vi "pt2line.vi"() -> ()   [LabVIEW 2012]
uses:
  <vilib>/Utility/file.llb/Read From Spreadsheet File (DBL).vi
  G_VEH.vi
  G_DATA.vi
panel:
  out "XY Graph":cluster{"Y":dbl[], "Y":dbl[]}[](graph)
  out "x":dbl[](array[numeric])
  out "y":dbl[](array[numeric])
  out "all rows":dbl[][](array[numeric]) format="%0.3f"
  out "path":dbl[][](array[numeric])=[[-255.216465, -224.019097, -197.334027, -175.46223, -152.92194, -136.088512, -102.998886, -54.784189, -7.516358, 50.306778, 91.062603, 97.084713, 93.1202, 88.769951, 86.75765, 81.589658, 76.301743, 66.513984, 61.367971, 45.319341, 14.450991, -36.946592, -51.800053, -55.664715, -72.629843, -125.329123, -146.219545, -155.532572, -155.231925, -148.150396, -135.052899, -119.630627, -107.638961, -104.13624, -102.377677, -84.094956, -59.779119, -30.298412, -1.547282, 2.854327, 6.657761, 10.459174, 3.511141, -26.30694, -73.476042, -111.842628, -118.995936, -116.921215, -102.705074, -88.210666, -83.464367, -86.343257, -102.617415, -107.759916], [-500.016381, -499.568356, -491.833583, -478.953387, -483.69293, -504.762747, -532.145235, -529.336413, -503.242034, -468.920949, -416.684928, -375.565995, -317.161413, -241.087674, -176.765644, 3.050236, 189.901281, 261.392787, 293.826989, 342.636657, 363.781536, 367.66991, 386.702929, 417.645918, 425.204416, 423.95351900000003, 421.057136, 404.578929, 377.734918, 362.899426, 359.271761, 354.312176, 342.051425, 318.167906, 262.459507, 222.699763, 207.938059, 194.431872, 156.064352, 93.448286, -37.349453, -127.219275, -172.925371, -232.424698, -322.447879, -394.422916, -407.829977, -419.760997, -428.914985, -435.912385, -441.894453, -447.061864, -442.947155, -438.571904], [-0.027619159683021918, 0.03119709854315155, 0.5801517623319503, 0.22974199850915422, -0.6985990286570105, -0.9293009663449048, -0.3629416523824042, 0.4364661436108174, 0.517269626400344, 0.6407274895950754, 1.202041727338265, 1.6238751525788475, 1.6374547962778776, 1.5888610615665095, 1.592488214998328, 1.6019260023104704, 1.6167108615873471, 1.7565325957017393, 1.6632287927306733, 2.2220223320446446, 2.8894133609140376, 2.6493725961179972, 1.7654388795036573, 2.1924575664831303, -3.124456663546736, -3.1171931962117276, -2.6388223143414686, -1.6335362194597147, -1.4505762061951697, -0.6355428134884025, 0.011046092972199223, -0.8136354408991358, -1.0376420447469035, -1.5493221762811478, -1.4668097598430623, -0.7797235340435182, -0.34848317538441986, -0.6205836790536368, -1.2605695601954436, -1.5525481966917887, -1.5407853718079607, -1.5350592142675334, -1.962733401760107, -2.0504512632483882, -2.048817660019718, -2.0492416975710537, -1.9356743047027372, -0.8584952334475433, -0.48041653333810286, -0.5197456398894826, -1.5337392732156923, -2.7467198900599588, 2.6204704682047826, 1.8591507266149765], [31.173097298848553, 26.913348647230613, 25.353412697049688, 20.868729331498855, 26.441054626560174, 41.739539871153646, 44.076619004466615, 53.86765552210779, 67.2303653094776, 63.8979451122852, 40.52548790718823, 58.532660795170074, 76.19455662891659, 64.34788473882465, 179.8856712687191, 186.9251021756951, 71.86540454258034, 32.82666676125214, 50.08261037391, 35.528613596596784, 50.7421338721755, 22.084837087831545, 31.10617534511584, 16.024654359701316, 52.71297713376437, 20.954867085973486, 16.10065419017421, 26.772345178567814, 15.577706313644756, 12.693639675564514, 15.366548203355588, 17.147584175475338, 22.348948287332743, 55.733315576213904, 41.44270545761075, 27.66988575085065, 32.320665344175666, 45.701271321041276, 60.97074789973921, 130.84536386325192, 89.94342098656917, 45.428662749114835, 66.37743516511998, 101.63171501074622, 81.55665134233071, 15.194986170689614, 10.405235150658818, 16.21963108303148, 16.08751584460026, 7.090579242568349, 5.057204630463252, 13.438898131348209, 6.638125580359146, 5.5967112451721], [-5.8005401539539816e-05, 9.377852292749824e-05, -0.0003539490410145481, -0.0005151318592905256, 0.0002235088483526294, 7.241195538871463e-05, 5.779564013674301e-05, -1.8487595581227712e-05, 1.3929893247701302e-05, 1.7883823331962755e-05, -6.307219310271541e-06, -3.006785820458783e-06, -3.158361707682015e-06, -4.455959476150721e-06, -1.3447632906964453e-07, 2.9815585665443266e-07, -8.766741899073422e-06, -1.884292765099321e-05, 5.227332045958214e-05, 0.00010206184484366903, -0.0002090696086899051, -0.0004240969337350295, 0.0005224443232844847, 0.0009379992925151037, -2.2273087775570565e-06, 0.00040741029669219764, 0.000878081447133453, 2.243486550958545e-05, 0.0009714058689747632, -0.00010628687919937756, -0.001450721296137834, -0.0006072609527100151, 0.0005250749412259796, 1.2471714391522846e-05, 7.415057073132304e-05, -2.273261670311925e-05, -9.32393806654143e-05, -4.2946907783804566e-05, 5.0825650117951696e-05, -6.200466545493865e-07, -1.439182072298954e-06, -3.398695471668847e-05, 1.5252474863614805e-05, 1.1327936413660916e-06, 3.1756015037854445e-06, 0.00019921266235668522, 0.003602519234707369, -0.0007715338539630026, -0.00024149961509246942, -0.0077472176379480995, -0.026326458891392825, 0.0013424692985958657, -0.0052589340705270805, 0.006322158195003703], [0.0031556466816350663, 0.007000305473368755, 0.007081592130884735, -0.011633188857604608, -0.013501739648532357, 0.002789755616338565, 0.007615128599941668, 0.002259298148540837, -0.0006628574354981043, 0.0031464701270773345, 0.005860008275585139, 0.0004271102423971235, 0.00011549228481064184, 0.0004920315551065756, 6.333068996620233e-05, -7.091040018093933e-05, 0.001887828967418721, -0.0002464591558994194, 0.0019568638083808615, 0.005669467066737969, 0.014127047728702505, -0.010632306877580938, -0.01851787629643413, 0.021532645124575006, 0.00024254157976403152, -0.0031037933454297188, 0.0242509159053178, 0.0021661853270953757, 0.006507376998295557, 0.031483511351547956, 0.0005688784121944422, 0.01141286265930296, -0.02999859746832826, -0.000514174890586656, 0.005111540169826646, 0.00924798537148707, 0.0004983016816273771, -0.004977023268713058, -0.0071133690367256456, 0.00016384500465515148, 0.00026579249686769287, -0.0026118495752822674, -0.002108545689237222, -0.00014446195942131656, -0.00040268393860428905, -0.0037956720386472208, 0.01973861823614979, 0.030671419641740347, 0.005791013618687458, -0.0014524476562737412, 0.013164858153403234, -0.0737354381001526, 0.006899030465801037, -0.11509378945355726], [38.56772665054293, 34.10122710666827, 26.360895547102693, 23.248175700753727, 29.730717905157913, 39.01961943373853, 35.89132192826281, 47.71217398816982, 57.90858834588869, 45.04837806650923, 45.023397984125, 55.69138253927084, 121.27440585459983, 115.14995278201658, 95.97898635414336, 70.75393092609372, 58.14850528330802, 51.4019530001095, 39.956574505496185, 29.096302609494554, 26.53820640294646, 24.390223251636094, 21.743799201903915, 19.26138503496554, 30.50353573698609, 21.27077286541254, 19.0585031837167, 25.129026995403002, 19.489391916263322, 19.431582182677115, 18.80975982660167, 20.00531960915423, 19.94900505227746, 42.81187756318914, 35.878512395055374, 35.84714285295909, 39.159064072751036, 39.767226518944916, 40.90211423753575, 70.67956774200063, 54.51331303545745, 46.36708296272543, 46.94893578363172, 49.859282930602404, 25.510322642962063, 17.573863589956417, 14.690372880063457, 19.751811771736076, 15.555267547891663, 11.64531096346214, 9.105731241174198, 12.727362742103542, 10.355560994042879, 10.246340620672186], [8.0, 8.0, 8.0, 8.0, 8.0, 8.0, 8.0, 8.0, 8.0, 8.0, 8.0, 8.0, 8.0, 8.0, 8.0, 8.0, 8.0, 8.0, 8.0, 8.0, 8.0, 8.0, 8.0, 8.0, 8.0, 8.0, 8.0, 8.0, 8.0, 8.0, 8.0, 8.0, 8.0, 8.0, 8.0, 8.0, 8.0, 8.0, 8.0, 8.0, 8.0, 8.0, 8.0, 8.0, 8.0, 8.0, 8.0, 8.0, 8.0, 8.0, 8.0, 8.0, 8.0, 7.0], [31.204058852732597, 28.127406314146373, 25.524943419248775, 23.8796266140581, 27.048823104873343, 43.547139107789874, 49.689415779153336, 54.01133245257729, 67.27694062901611, 67.16724847514878, 41.8665010656562, 58.54003483830677, 76.20311853440715, 64.35421763760496, 179.89092543127825, 186.9265371123329, 72.21661150390257, 32.848390437875494, 52.05802860970812, 38.194925547149126, 51.965901750979654, 24.96423893800446, 31.549942906621784, 19.41539366339203, 52.714282942301445, 21.246819679907066, 19.80906941992803, 26.876209247634286, 16.893295353316248, 13.835823225042914, 16.759094394266835, 17.17869437382284, 24.40836723381224, 55.74634624174131, 44.70380948692326, 28.669982813187747, 32.52643709968685, 48.80312149263486, 63.037893472912245, 130.85405975088685, 89.95111358558907, 46.59230684804797, 66.57723351081263, 101.63265494652278, 81.56317928744686, 15.197155542415661, 12.783099305960778, 17.01487652979347, 16.09664609983255, 7.976923256658123, 6.372558984688654, 17.294923976288672, 6.853888590460845, 6.223964924900602], [46.768692163461566, 38.5385461380969, 35.46865514741364, 27.040309600418997, 29.730717905157913, 46.661652675810544, 39.037663412421914, 47.71217398816982, 69.74861693251641, 57.88915791495063, 45.023397984125, 55.69138253927084, 128.13977263212485, 121.26512901647978, 115.14018249812098, 95.96726432262606, 70.7380289621812, 58.12915504875507, 51.380062010298865, 39.92840900725143, 29.057612140448136, 27.427658055934497, 25.431465225996796, 21.79307468418614, 31.179550095454193, 30.466632441936177, 21.217817315354946, 32.255432660709424, 25.08421809116186, 19.431582182677115, 23.729859655200077, 23.713687690037577, 19.94900505227746, 55.54186183134492, 42.78559173589523, 35.84714285295909, 46.88736527093776, 39.767226518944916, 40.90211423753575, 78.99805189964593, 70.66364904387021, 54.49267196628217, 46.94893578363172, 69.0683198565055, 49.83671432139203, 25.46618466098998, 17.509730921227597, 19.751811771736076, 24.53346445960561, 15.482775863219398, 11.548301441675308, 12.727362742103542, 16.098646796948746, 10.246340620672186], [46.768692163461566, 35.388795108509086, 26.921219169168285, 24.020374908691828, 50.03732710858249, 40.231702958175575, 37.537393237331884, 76.87062876466402, 69.74861693251641, 53.33805515919421, 45.023397984125, 130.69013395633164, 128.13977263212485, 121.26512901647978, 115.14018249812098, 95.96726432262606, 70.7380289621812, 58.12915504875507, 43.919351337089566, 35.735869499979415, 40.367375263663774, 25.226427811403333, 32.11867508853556, 20.007932871216823, 45.415162967737004, 30.466632441936177, 19.84330317637312, 34.99886048851328, 21.260411525619922, 25.422143122170613, 19.357930602736715, 27.807022960628544, 49.288310479939746, 55.54186183134492, 38.49446918699541, 35.84714285295909, 39.159064072751036, 42.695776435820115, 80.99729421186991, 88.66266180749345, 70.66364904387021, 47.888528946368474, 78.01370244811137, 69.0683198565055, 49.83671432139203, 25.46618466098998, 15.1442959932323, 28.991581428930765, 24.53346445960561, 12.748651537375247, 9.38074110508569, 22.17115712782233, 16.098646796948746, 28.08043202008495], [38.56772665054293, 35.49560087043334, 26.360895547102693, 29.768533541310575, 46.68575618457934, 39.0664711146902, 47.2064777912347, 69.76474442011407, 57.90858834588869, 45.04837806650923, 55.25875576858096, 128.14855180692754, 121.27440585459983, 115.14995278201658, 95.97898635414336, 70.75393092609372, 58.14850528330802, 51.4019530001095, 39.956574505496185, 29.096302609494554, 26.53820640294646, 25.47566343350262, 21.761470986994677, 30.400071449600134, 30.50353573698609, 21.27077286541254, 31.502586163696193, 25.129026995403002, 19.489391916263322, 23.77722101629017, 22.67904215198627, 20.00531960915423, 55.56211313201802, 42.81187756318914, 35.878512395055374, 46.3726753810148, 39.159064072751036, 40.92960969358078, 78.69366050663011, 70.67956774200063, 54.51331303545745, 46.434928342250956, 69.08460615651495, 49.859282930602404, 25.510322642962063, 17.573863589956417, 19.808686952854117, 24.579277425605213, 15.555267547891663, 11.64531096346214, 12.815452520728028, 16.16837744332587, 10.355560994042879, 35.0], [0.1, 10.4, 23.700000000000003, 6.9, 12.5, 24.700000000000003, 5.2, 7.7, 0.1, 22.500000000000004, 0.1, 29.300000000000004, 0.1, 0.1, 0.1, 0.1, 0.1, 0.1, 31.400000000000006, 14.1, 10.1, 7.5, 4.3, 3.4000000000000004, 2.4000000000000004, 0.1, 2.6, 0.5, 7.8999999999999995, 9.7, 8.4, 0.6, 14.500000000000004, 0.1, 15.5, 0.1, 32.320665344175666, 14.0, 33.10000000000001, 3.5000000000000004, 0.1, 29.900000000000006, 8.2, 0.1, 0.1, 0.1, 3.5000000000000004, 6.4, 0.1, 3.5000000000000004, 2.1, 6.4, 0.1, 4.7]]
  out "error out":errorcluster
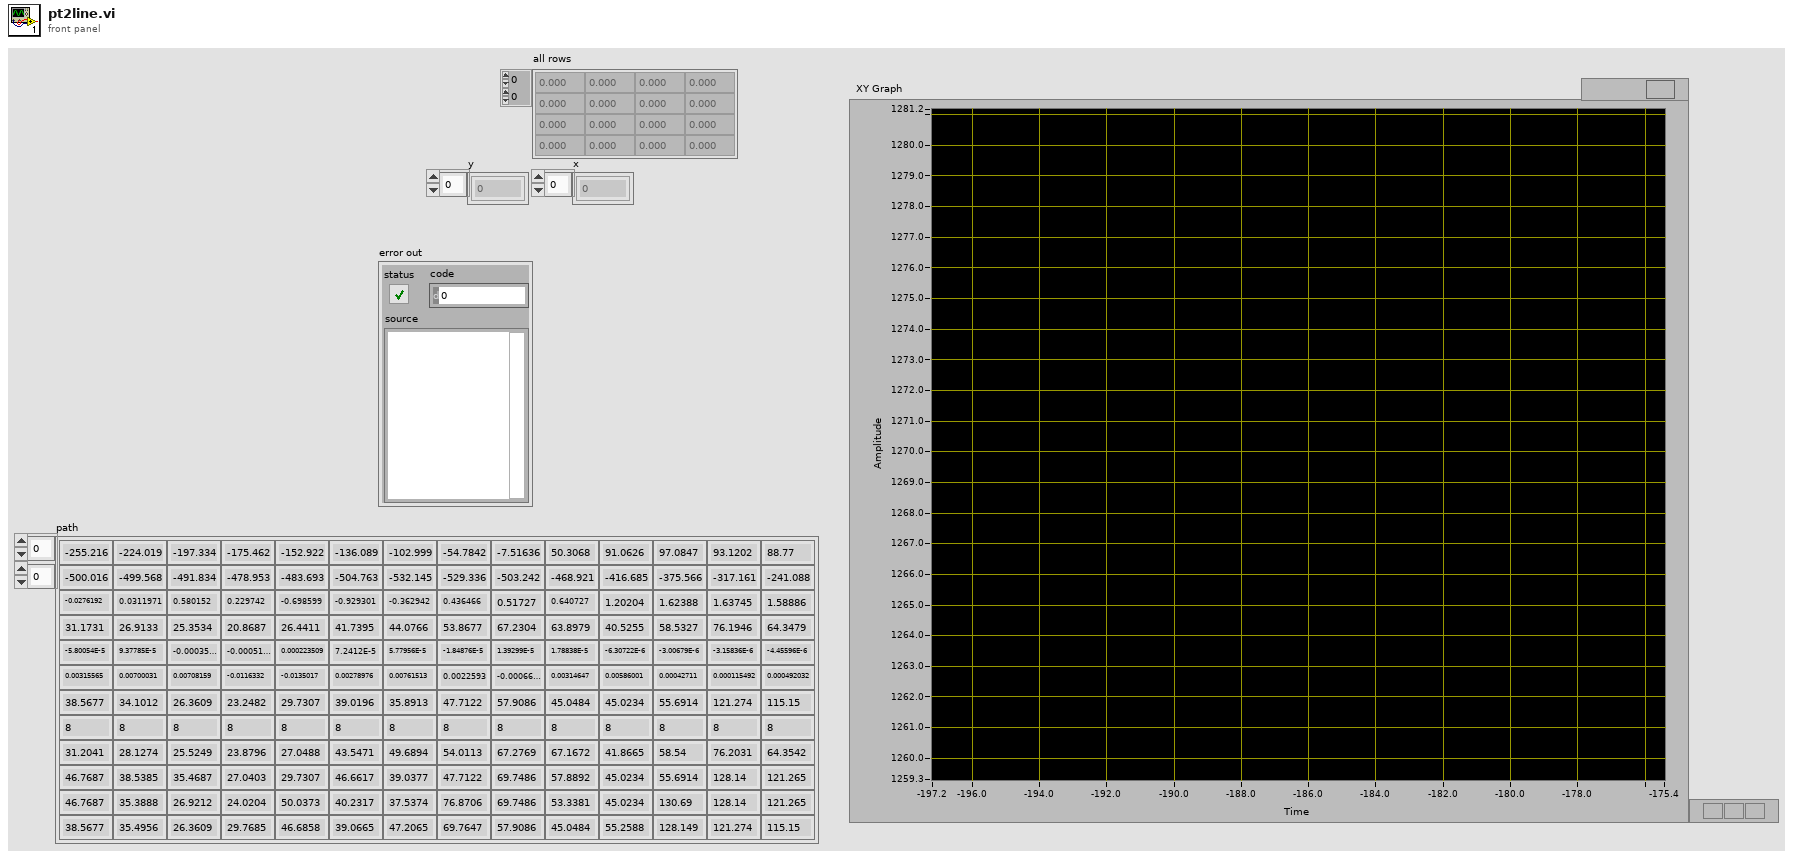
[diagram p1: front panel]
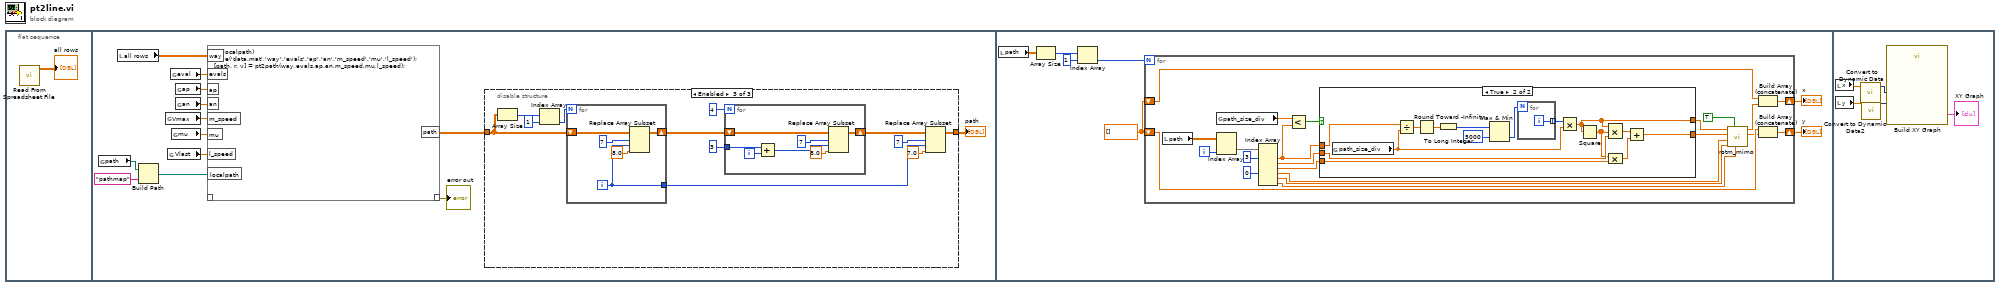
[diagram p0: block diagram]
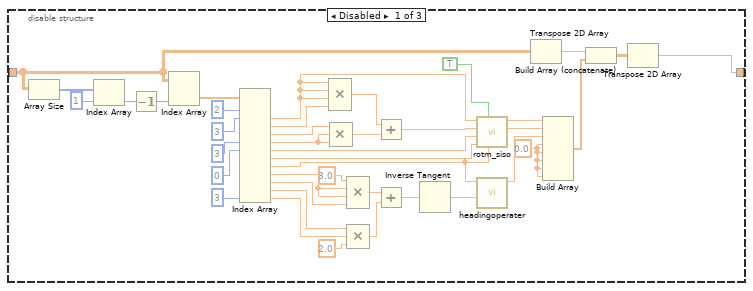
[diagram p2: hidden frame]
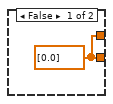
[diagram p4: hidden frame]
diagram:
  n1 = flat-sequence {
    frame #0 {
      n2 = call-poly <vilib>:"Read From Spreadsheet File.vi"() -> ("all rows"=→"all rows":dbl[][])  [unwired: 7 in, 4 out]
    }
    frame #1 {
      n3 = global read "G_DATA.vi" "path"() -> (w7:path)
      n4 = local read "all rows"() -> (w3:dbl[][])
      n5 = Build Path(base path=w7, name or relative path="pathmap") -> (appended path=w5:path)
      n6 = global read "G_VEH.vi" "Vmax"() -> (w10:dbl)
      n7 = global read "G_VEH.vi" "Vlast"() -> (w8:dbl)
      n8 = global read "G_VEH.vi" "eval"() -> (w13:dbl)
      n9 = global read "G_VEH.vi" "mu"() -> (w9:dbl)
      n10 = global read "G_VEH.vi" "ap"() -> (w12:dbl)
      n11 = global read "G_VEH.vi" "an"() -> (w11:dbl)
      n12 = script code="cd(localpath)\nsave('data.mat','way','evals','ap','an','m_speed','mu','l_speed');\n[path, r, v] = pt2path(way,evals,ap,an,m_speed,mu,l_speed);" ("Script Node")("way"=w3, "evals"=w13, "ap"=w12, "an"=w11, "m_speed"=w10, "mu"=w9, "l_speed"=w8, "localpath"=w5) -> ("??"=→"error out":errorcluster, "path"=w14:dbl[][])  [unwired: 1 in]
      n13 = disable-structure shown="Enabled" {
        disable-tunnel: w14 -> [w18 w55 w67]
        disable-tunnel: [w15 w55 w60] -> w2
        frame Disabled {
          w20 = 0.0 ("element")
          n14 = Array Size(array=w18) -> (size(s)=w54:i32[])
          n15 = Index Array(array=w54, index=1) -> (element=w52:i32)
          n16 = Decrement(x=w52) -> (x-1=w51:i32)
          n17 = Index Array(array=w18, index (col)=w51) -> (element=w24:dbl[])  [unwired: 1 in]
          n18 = Index Array(array=w24, index #1=2 ("index"), index #2=3 ("index"), index #5=3 ("index"), index #6=0 ("index"), index #12=3 ("index")) -> (element #2=w36:dbl, element #3=w37:dbl, element #4=w38:dbl, element #5=w40:dbl, element #6=w43:dbl, element #7=w44:dbl, element #8=w50:dbl, element #9=w45:dbl, element #10=w46:dbl, element #11=w47:dbl, element #12=w49:dbl)  [unwired: 7 in, 1 out]
          n19 = Compound Arithmetic op=MULTIPLY(w36, w36, w36, w37) -> (w34:dbl)
          n20 = Compound Arithmetic op=MULTIPLY(w38, w40, w40) -> (w33:dbl)
          n21 = Compound Arithmetic op=MULTIPLY(3.0 ("value"), w45, w45, w46) -> (w31:dbl)
          n22 = Compound Arithmetic op=MULTIPLY(w47, w49, 2.0 ("value")) -> (w32:dbl)
          n23 = Add(x=w34, y=w33) -> (x+y=w26:dbl)
          n24 = Add(x=w31, y=w32) -> (x+y=w28:dbl)
          n25 = Inverse Tangent(1:w28) -> (0:w27:dbl)
          n26 = call "rotm_siso.vi"("angle[rad]"=w50, "reverse"=TRUE, "y0"=w44, "x0"=w43, "y"=w26, "x"=w36) -> ("y'"=w22:dbl, "x'"=w23:dbl)  [unwired: 4 in]
          n27 = call "headingoperater.vi"("h1"=w27, "h2"=w50) -> ("h2+h1"=w21:dbl)  [unwired: 8 in, 1 out]
          n28 = Transpose 2D Array(2D array=w18) -> (transposed array=w17:dbl[][])
          n29 = Build Array(w23, w22, w21, w20, w20, w20, w20, w20) -> (w19:dbl[])
          n30 = Build Array (concatenate)(w17, w19) -> (w16:dbl[][])
          n31 = Transpose 2D Array(2D array=w16) -> (transposed array=w15:dbl[][])
        }
        frame Disabled {
        }
        frame Enabled {
          n32 = Array Size(array=w67) -> (size(s)=w66:i32[])
          n33 = Index Array(array=w66, index=1) -> (element=w64:i32)
          n34 = for {
            N: w64 -> [_]
            shift-right: [w76] -> w59
            shift-left: w67 -> [w79]
            tunnel: [w75] -> w63
            i -> [w75]
            n35 = Replace Array Subset(array=w79, new element=8.0 ("new element/subarray"), index (row)=7 ("disabled index (row)"), index (col)=w75) -> (w76:dbl[][])
          }
          n36 = for {
            N: 4 -> [_]
            shift-right: [w71] -> w58
            shift-left: w59 -> [w74]
            tunnel: 3 -> [w70]
            i -> [w69]
            n37 = Add(x=w70, y=w69) -> (x+y=w68:i32)
            n38 = Replace Array Subset(array=w74, new element=8.0 ("new element/subarray"), index (row)=7 ("disabled index (row)"), index (col)=w68) -> (w71:dbl[][])
          }
          n39 = Replace Array Subset(array=w58, new element=7.0 ("new element/subarray"), index (row)=7 ("disabled index (row)"), index (col)=w63) -> (w60:dbl[][])
        }
      }
      "path" <- w2
    }
    frame #2 {
      w84 = dbl[] []
      n40 = local read "path"() -> (w83:dbl[][])
      n41 = Array Size(array=w83) -> (size(s)=w85:i32[])
      n42 = Index Array(array=w85, index=1) -> (element=w80:i32)
      n43 = for {
        N: w80 -> [_]
        shift-right: [w92] -> w81
        shift-left: w84 -> [w94]
        shift-right: [w89] -> w82
        shift-left: w84 -> [w91]
        i -> [w88]
        n44 = local read "path"() -> (w87:dbl[][])
        n45 = global read "G_VEH.vi" "path_size_div"() -> (w103:dbl)
        n46 = Index Array(array=w87, index (col)=w88) -> (element=w108:dbl[])  [unwired: 1 in]
        n47 = Index Array(array=w108, index #1=3 ("index"), index #4=0 ("index")) -> (element #1=w102:dbl, element #2=w105:dbl, element #3=w104:dbl, element #4=w97:dbl, element #5=w96:dbl, element #6=w95:dbl)  [unwired: 4 in]
        n48 = Less?(x=w103, y=w102) -> (x < y?=w106:bool)
        n49 = case shown="True" w106 {
          tunnel: w102 -> [_ w124]
          tunnel: w105 -> [_ w119]
          tunnel: w104 -> [_ w118]
          tunnel: [w109 w114] -> w101
          tunnel: [w109 w113] -> w100
          frame False {
            w109 = dbl[] [0.0]
          }
          frame True {
            n50 = global read "G_VEH.vi" "path_size_div"() -> (w120:dbl)
            n51 = Divide(x=w124, y=w120) -> (x/y=w123:dbl)
            n52 = Round Toward -Infinity(1:w123) -> (0:w122:dbl)
            n53 = To Long Integer(number=w122) -> (32bit integer=w111:i32)
            n54 = Max & Min(x=w111, y=5000) -> (min(x,y)=w110:i32)  [unwired: 1 out]
            n55 = for {
              N: w110 -> [_]
              tunnel: [w125] -> w121 mode=indexing
              i -> [w125]
            }
            n56 = Multiply(x=w121, y=w120) -> (x*y=w114:dbl[])
            n57 = Square(x=w114) -> (x^2=w115:dbl[])
            n58 = Compound Arithmetic op=MULTIPLY(w114, w115, w119) -> (w117:dbl[])
            n59 = Compound Arithmetic op=MULTIPLY(w115, w118) -> (w116:dbl[])
            n60 = Add(x=w117, y=w116) -> (x+y=w113:dbl[])
          }
        }
        n61 = call "rotm_mimo.vi"("angle[rad]"=w95, "reverse"=TRUE, "y0"=w96, "x0"=w97, "y"=w100, "x"=w101) -> ("Y"=w90:dbl[], "X"=w93:dbl[])  [unwired: 2 in, 2 out]
        n62 = Build Array (concatenate)(w94, w93) -> (w92:dbl[])
        n63 = Build Array (concatenate)(w91, w90) -> (w89:dbl[])
      }
      "y" <- w82
      "x" <- w81
    }
    frame #3 {
      n64 = local read "x"() -> (w129:dbl[])
      n65 = local read "y"() -> (w127:dbl[])
      n66 = call "Convert to Dynamic Data"("Array"=w129) -> ("Dynamic Data Type"=w128:dynamicdata)  [unwired: 3 in]
      n67 = call "Convert to Dynamic Data2"("Array"=w127) -> ("Dynamic Data Type"=w126:dynamicdata)  [unwired: 3 in]
      n68 = call "Build XY Graph"("Y Input"=w126, "X Input"=w128) -> ("XY Graph"=→"XY Graph":cluster{"Y":dbl[], "Y":dbl[]}[])  [unwired: 3 in, 6 out]
    }
  }
